vi "Node - PXImc Intial Handshaking.vi"(5 "Reader Buffer Size In":u64, 6 "Data In":u32[](array[numeric]), 7 "Connection Timeout (s)":dbl, 8 "error in (no error)":errorcluster, 9 "Reader Conn ID":u16, 10 "Writer Conn ID":u16, 11 "Resource Name In":string) -> (0 "error out":errorcluster)   [LabVIEW 2016, in "PXImc Router.lvlib"]
uses:
  PXImc Router.lvlib
  <vilib>/pximc/Initialize Writer Session (U32).vi
  <vilib>/pximc/Initialize Reader Session (U32).vi
  <vilib>/pximc/Connect (U32).vi
  <vilib>/pximc/Write (U32).vi
  <vilib>/pximc/Read (U32).vi
  <vilib>/pximc/nipximc.lvlib
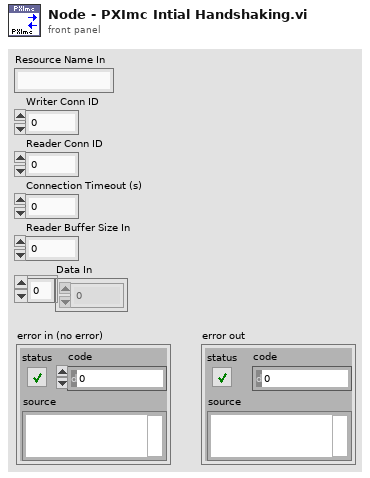
[diagram p1: front panel]
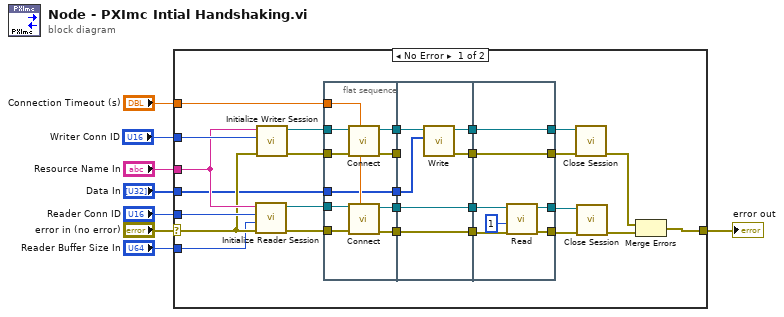
[diagram p0: block diagram]
diagram:
  n1 = case shown="No Error" "error in (no error)" {
    selector: "error in (no error)" -> [w12 w59]
    tunnel: "Writer Conn ID" -> [w27 _]
    tunnel: "Reader Conn ID" -> [w26 _]
    tunnel: "Reader Buffer Size In" -> [w9 _]
    tunnel: "Resource Name In" -> [w25 _]
    tunnel: "Connection Timeout (s)" -> [w24 _]
    tunnel: [w19 w59] -> w3
    tunnel: "Data In" -> [w11 _]
    frame No Error {
      n2 = call-poly <vilib>:"Initialize Reader Session.vi"("error in (no error)"=w12, "buffer size"=w9, "writer's connection id (1)"=w26, "interface"=w25) -> ("error out"=w16:errorcluster, "session out"=w15:refnum<k21>)  [unwired: 6 in]
      n3 = call-poly <vilib>:"Initialize Writer Session.vi"("error in (no error)"=w12, "connection id (1)"=w27, "interface"=w25) -> ("error out"=w14:errorcluster, "session out"=w13:refnum<k21>)  [unwired: 7 in]
      n4 = flat-sequence {
        tunnel: w13 -> [w45]
        tunnel: w14 -> [w44]
        tunnel: w15 -> [w41]
        tunnel: w16 -> [w40]
        tunnel: [w43] -> w35
        tunnel: [w42] -> w34
        tunnel: [w39] -> w33
        tunnel: [w38] -> w32
        tunnel: w24 -> [w37]
        tunnel: w11 -> [w36]
        tunnel: [w36] -> w10
        tunnel: w35 -> [w49]
        tunnel: w34 -> [_]
        tunnel: w33 -> [w51]
        tunnel: w32 -> [w50]
        tunnel: [w48] -> w31
        tunnel: [w47] -> w30
        tunnel: [w51] -> w29
        tunnel: [w50] -> w28
        tunnel: w10 -> [w46]
        tunnel: [w57] -> w23
        tunnel: [w58] -> w22
        tunnel: w31 -> [w58]
        tunnel: w30 -> [w57]
        tunnel: w29 -> [w55]
        tunnel: w28 -> [w56]
        tunnel: [w54] -> w21
        tunnel: [w53] -> w20
        frame #0 {
          n5 = call-poly <vilib>:"Connect.vi"("timeout in seconds (-1)"=w37, "error in (no error)"=w44, "session in"=w45) -> ("error out"=w42:errorcluster, "session out"=w43:refnum<k21>)  [unwired: 7 in]
          n6 = call-poly <vilib>:"Connect.vi"("timeout in seconds (-1)"=w37, "error in (no error)"=w40, "session in"=w41) -> ("error out"=w39:errorcluster, "session out"=w38:refnum<k21>)  [unwired: 7 in]
        }
        frame #1 {
          n7 = call-poly <vilib>:"Write.vi"("data"=w46, "session in"=w49) -> ("error out"=w47:errorcluster, "session out"=w48:refnum<k21>)  [unwired: 7 in, 1 out]
        }
        frame #2 {
          n8 = call-poly <vilib>:"Read.vi"("error in (no error)"=w55, "number of elements"=1, "session in"=w56) -> ("error out"=w54:errorcluster, "session out"=w53:refnum<k21>)  [unwired: 6 in, 1 out]
        }
      }
      n9 = call <vilib>:"Close Session.vi"("error in (no error)"=w23, "session in"=w22) -> ("error out"=w17:errorcluster)  [unwired: 9 in]
      n10 = call <vilib>:"Close Session.vi"("error in (no error)"=w21, "session in"=w20) -> ("error out"=w18:errorcluster)  [unwired: 9 in]
      n11 = Merge Errors(w17, w18) -> (w19:errorcluster)
    }
    frame Error {
    }
  }
  "error out" <- w3
